vi "Create Base.vi"(9 "jettl":refnum<class "jettl.lvclass">, 10 "Self Alias":string) -> (0 "error out":errorcluster)   [LabVIEW 2021, in "jettl.lvlib" / "Base Event.lvlib"]
uses:
  Base Event.lvlib
  Base Event/Base Event.lvclass
  jettl/jettl.lvclass
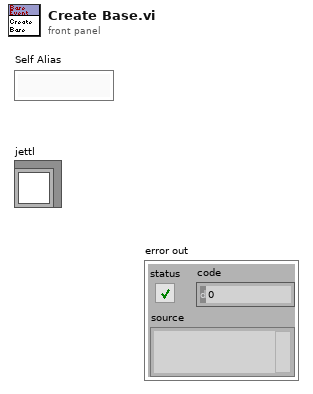
[diagram p1: front panel]
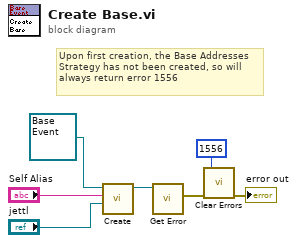
[diagram p0: block diagram]
diagram:
  # "Upon first creation, the Base Addresses Strategy has not been created, so will always return error 1556"
  n1 = call-dynamic "Create.vi"("jettl"="jettl", "Self Alias"="Self Alias", "Base Event in"=refnum<class "Base Event.lvclass"> refnum ("jettl.lvlib:Base Event.lvlib:Base Event.lvclass")) -> ("Base Event out"=w7:refnum<class "Base Event.lvclass">)  [unwired: 8 in]
  n2 = call-dynamic "Get Error.vi"("Base Event in"=w7) -> ("Error"=w4:errorcluster)  [unwired: 10 in]
  n3 = call <vilib>:"Clear Errors.vi"("error in (no error)"=w4, "specific error code to clear (0: all)"=1556) -> ("error out"=→"error out":errorcluster)  [unwired: 4 in, 1 out]
